vi "Configure Trigger In.vi"(8 "error in (no error)":errorcluster, 9 "External Trigger Slope (T: Positive)":bool, 10 "Trigger Source (0:Immediate)":enum16{"Immediate", "External", "Bus"}(ring), 11 "VISA resource name":refnum<visa-resource-name>) -> (0 "error out":errorcluster, 3 "VISA resource name out":refnum<visa-resource-name>)   [LabVIEW 2017, in "Keithley 3390.lvlib"]
doc: "Configures the function generator's input trigger. Trigger is used with burst mode to initiate a burst cycle."
uses:
  Keithley 3390.lvlib
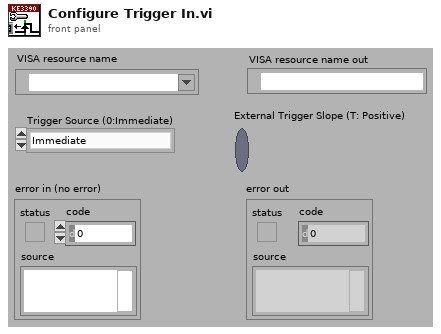
[diagram p1: front panel]
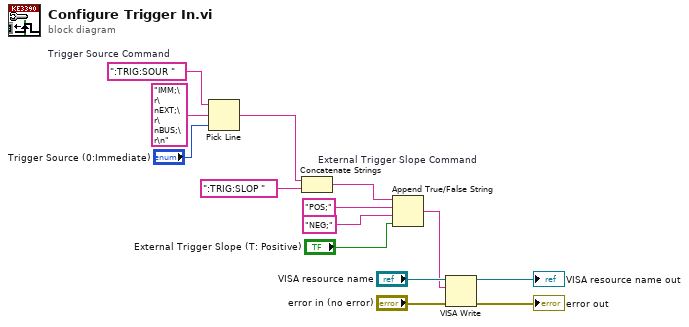
[diagram p0: block diagram]
diagram:
  w3 = ":TRIG:SOUR "  # Trigger Source Command
  w6 = ":TRIG:SLOP "  # External Trigger Slope Command
  n1 = Pick Line(string ("")=w3, multi-line string="IMM;\r\nEXT;\r\nBUS;\r\n" ("options"), line index="Trigger Source (0:Immediate)") -> (output string=w7:string)
  n2 = Concatenate Strings(w7, w6) -> (w5:string)
  n3 = Append True/False String(1:"External Trigger Slope (T: Positive)", 2:"NEG;" ("false string"), 3:"POS;" ("true string"), 4:w5) -> (0:w4:string)
  n4 = VISA Write(VISA resource name="VISA resource name", write buffer=w4, error in (no error)="error in (no error)") -> (VISA resource name out=→"VISA resource name out":refnum<visa-resource-name>, error out=→"error out":errorcluster)  [unwired: 1 out]
